vi "PathPlanner_Path_RePlan_Worker2.vi"(4 "StartingPoseTranslation":T1 {"Y" format="%14.3f"; "X" format="%14.3f"}, 5 "in PathPlannerPath":T2 {"AllPoints"."HolonomicRotation"."SIN" format="%13.4f"; "AllPoints"."HolonomicRotation"."COS" format="%13.4f"; "AllPoints"."HolonomicRotation"."VALUE" format="%13.4f"; "AllPoints"."Position"."Y" format="%14.3f"; "AllPoints"."Position"."X" format="%14.3f"; "GoalEndState"."Rotation"."SIN" format="%13.4f"; "GoalEndState"."Rotation"."COS" format="%13.4f"; "GoalEndState"."Rotation"."VALUE" format="%13.4f"; "EventMarkers"."lastRobotPos"."Y" format="%14.3f"; "EventMarkers"."lastRobotPos"."X" format="%14.3f"; "EventMarkers"."markerPos"."Y" format="%14.3f"; "EventMarkers"."markerPos"."X" format="%14.3f"; "RotationTargets"."target"."SIN" format="%13.4f"; "RotationTargets"."target"."COS" format="%13.4f"; "RotationTargets"."target"."VALUE" format="%13.4f"; "PreviewStartingRotation"."SIN" format="%13.4f"; "PreviewStartingRotation"."COS" format="%13.4f"; "PreviewStartingRotation"."VALUE" format="%13.4f"; "BezierPoints"."Y" format="%14.3f"; "BezierPoints"."X" format="%14.3f"}, 6 "robotNextCtrl":T1 {"Y" format="%14.3f"; "X" format="%14.3f"}, 7 "NumPtsMinusOne":i32, 9 "robotNextCtrl_NULL":bool, 10 "ComparePoint":T1 {"Y" format="%14.3f"; "X" format="%14.3f"}, 11 "ClosestDist":dbl) -> (2 "Error":bool, 3 "Replanned Path":T2 {"AllPoints"."HolonomicRotation"."SIN" format="%13.4f"; "AllPoints"."HolonomicRotation"."COS" format="%13.4f"; "AllPoints"."HolonomicRotation"."VALUE" format="%13.4f"; "AllPoints"."Position"."Y" format="%14.3f"; "AllPoints"."Position"."X" format="%14.3f"; "GoalEndState"."Rotation"."SIN" format="%13.4f"; "GoalEndState"."Rotation"."COS" format="%13.4f"; "GoalEndState"."Rotation"."VALUE" format="%13.4f"; "EventMarkers"."lastRobotPos"."Y" format="%14.3f"; "EventMarkers"."lastRobotPos"."X" format="%14.3f"; "EventMarkers"."markerPos"."Y" format="%14.3f"; "EventMarkers"."markerPos"."X" format="%14.3f"; "RotationTargets"."target"."SIN" format="%13.4f"; "RotationTargets"."target"."COS" format="%13.4f"; "RotationTargets"."target"."VALUE" format="%13.4f"; "PreviewStartingRotation"."SIN" format="%13.4f"; "PreviewStartingRotation"."COS" format="%13.4f"; "PreviewStartingRotation"."VALUE" format="%13.4f"; "BezierPoints"."Y" format="%14.3f"; "BezierPoints"."X" format="%14.3f"})   [LabVIEW 2019, in "PathPlanner24.lvlib"]
doc: "Replan path worker 1\n\nNOT COMPLETE. DONT USE."
uses:
  PathPlanner24.lvlib
  TypeDef/PathPlannerPath.ctl
  <vilib>/Rock Robotics/WPI/ThirdParty/JAS_Junk/TrajLib/TypeDef/TRANSLATION2D.ctl
  <vilib>/Rock Robotics/WPI/ThirdParty/JAS_Junk/TrajLib/TypeDef/ROTATION2D.ctl
  TypeDef/PathPlannerRotationTarget.ctl
  TypeDef/PathPlannerConstraintsZone.ctl
  TypeDef/PathPlannerPathConstraints.ctl
  TypeDef/PathPlannerEventMarker.ctl
  TypeDef/PathPlannerCommandUtil.ctl
  ENum/PathPlanner_CommandUtilType_ENUM.ctl
  TypeDef/PathPlannerGoalEndState.ctl
  TypeDef/PathPlannerPathPoint.ctl
  <vilib>/Rock Robotics/WPI/ThirdParty/JAS_Junk/TrajLib/Translation2d_Create.vi
  <vilib>/Rock Robotics/WPI/ThirdParty/JAS_Junk/TrajLib/Translation2d_GetXY.vi
  <vilib>/Rock Robotics/WPI/ThirdParty/JAS_Junk/TrajLib/Rotation2d_CreateXY.vi
  <vilib>/Rock Robotics/WPI/ThirdParty/JAS_Junk/TrajLib/Rotation2d_GetAngleCosSin.vi
  <vilib>/Rock Robotics/WPI/ThirdParty/JAS_Junk/TrajLib/Util_CalcDist.vi
  <vilib>/Rock Robotics/WPI/ThirdParty/JAS_Junk/TrajLib/Trajectory_Library.lvlib
panel:
  # "NOT DONE"
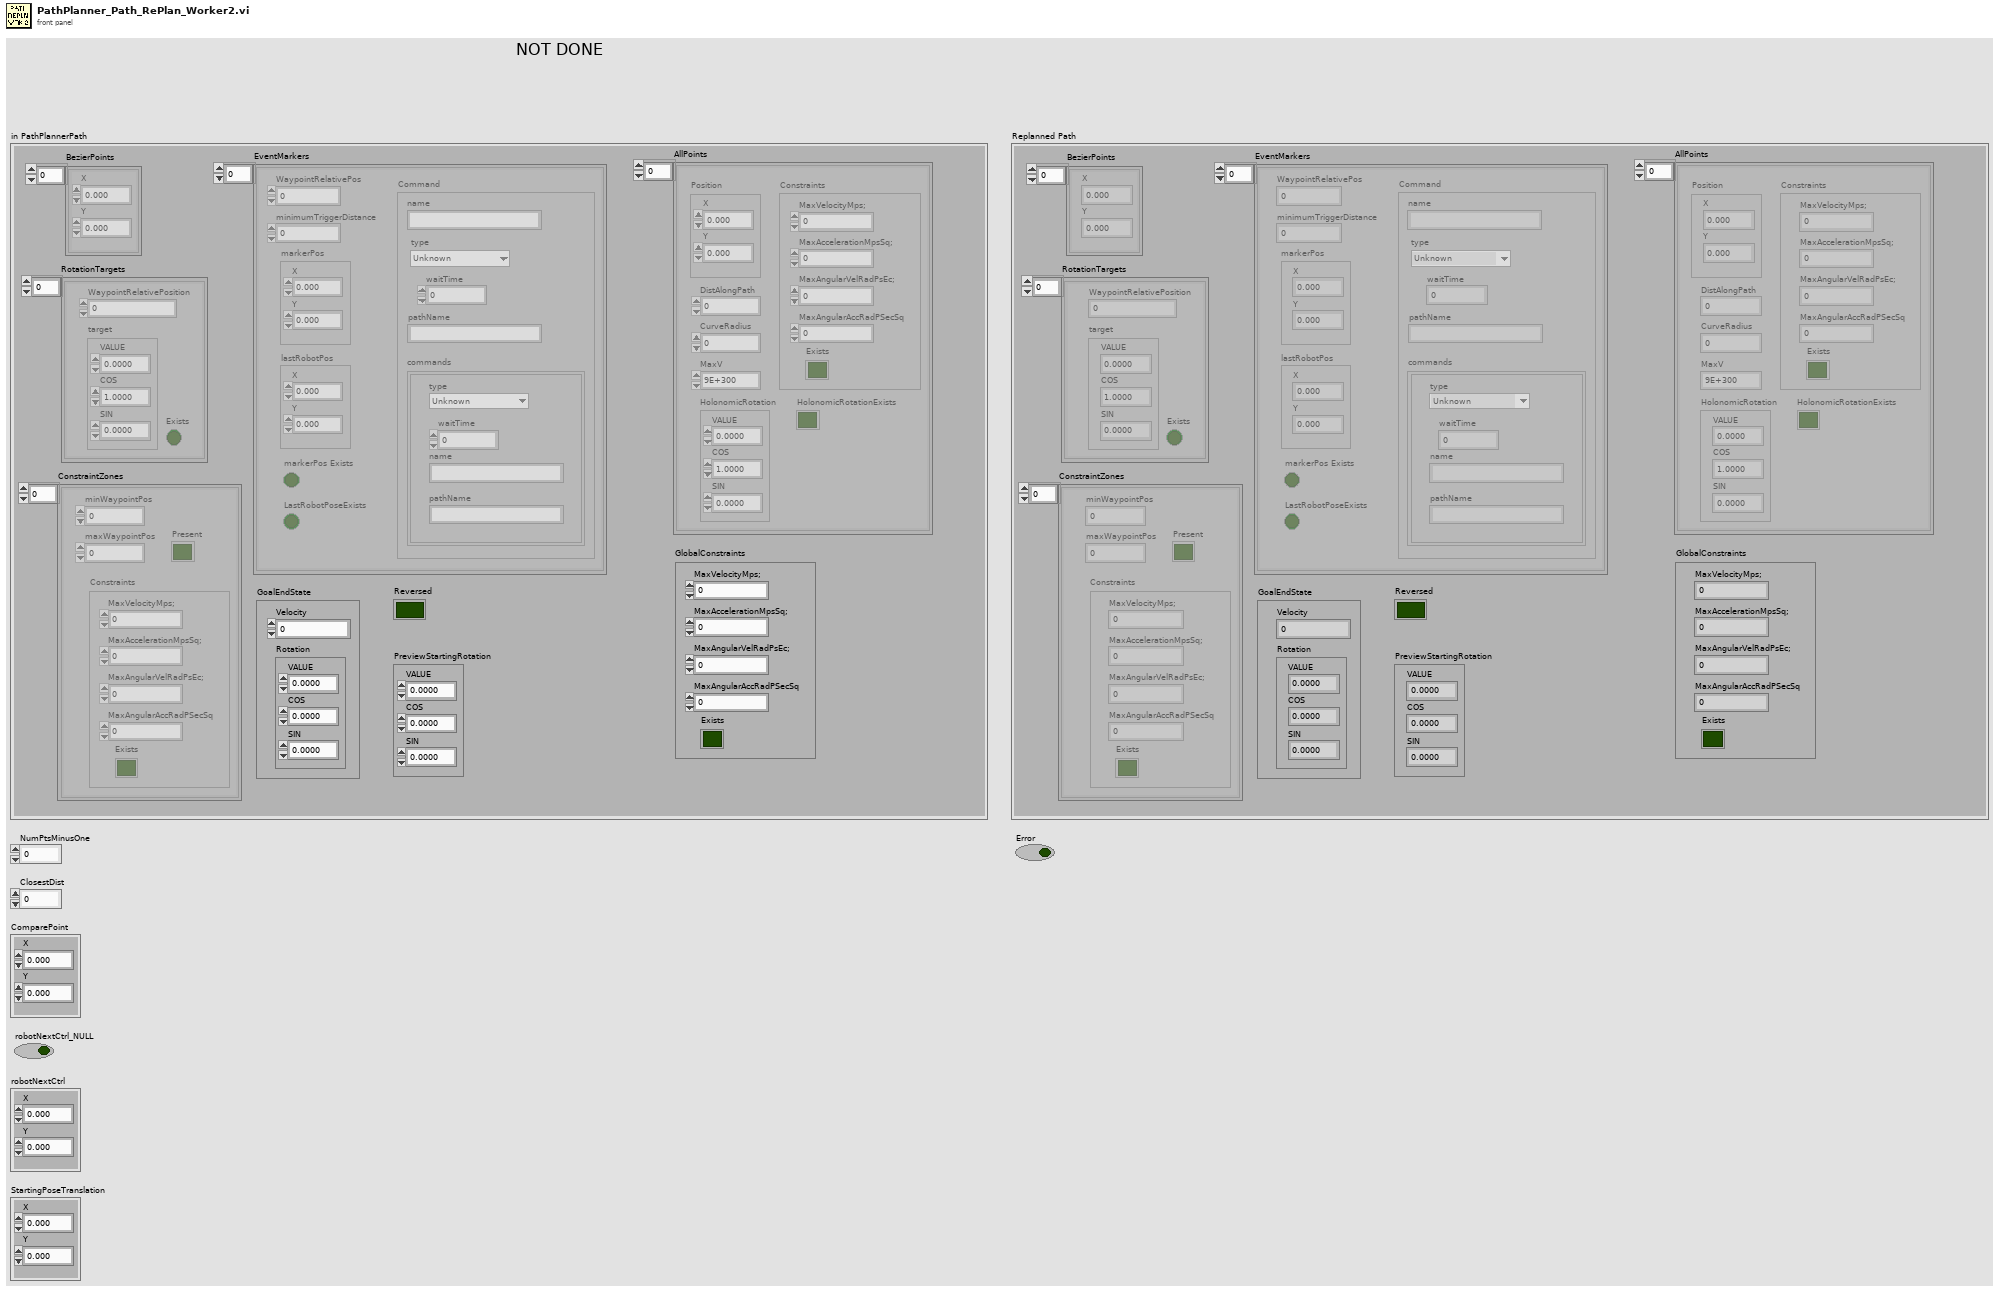
[diagram p1: front panel]
types:
  T1 = typedef "Trajectory_Library.lvlib/TRANSLATION2D.ctl" = cluster{"X":dbl, "Y":dbl}
  T2 = typedef "PathPlanner24.lvlib/PathPlannerPath.ctl" = cluster{"BezierPoints":T1[], "PreviewStartingRotation":T3, "Reversed":bool, "RotationTargets":T4[], "ConstraintZones":T5[], "EventMarkers":T7[], "GlobalConstraints":T6, "GoalEndState":T10, "AllPoints":T11[]}
  T3 = typedef "Trajectory_Library.lvlib/ROTATION2D.ctl" = cluster{"VALUE":dbl, "COS":dbl, "SIN":dbl}
  T4 = typedef "PathPlanner24.lvlib/PathPlannerRotationTarget.ctl" = cluster{"target":T3, "WaypointRelativePosition":dbl, "Exists":bool}
  T5 = typedef "PathPlanner24.lvlib/PathPlannerConstraintsZone.ctl" = cluster{"minWaypointPos":dbl, "maxWaypointPos":dbl, "Constraints":T6, "Present":bool}
  T6 = typedef "PathPlanner24.lvlib/PathPlannerPathConstraints.ctl" = cluster{"MaxVelocityMps;":dbl, "MaxAccelerationMpsSq;":dbl, "MaxAngularVelRadPsEc;":dbl, "MaxAngularAccRadPSecSq":dbl, "Exists":bool}
  T7 = typedef "PathPlanner24.lvlib/PathPlannerEventMarker.ctl" = cluster{"WaypointRelativePos":dbl, "minimumTriggerDistance":dbl, "markerPos":T1, "lastRobotPos":T1, "Command":T8, "markerPos Exists":bool, "LastRobotPoseExists":bool}
  T8 = typedef "PathPlanner24.lvlib/PathPlannerCommandUtil.ctl" = cluster{"waitTime":dbl, "name":string, "pathName":string, "commands":cluster{"type":T9, "waitTime":dbl, "name":string, "pathName":string}[], "type":T9}
  T9 = typedef "PathPlanner24.lvlib/PathPlanner_CommandUtilType_ENUM.ctl" = enum16{"Unknown", "Wait", "Named", "Path", "Sequential", "Parallel", "Race", "Deadline"}
  T10 = typedef "PathPlanner24.lvlib/PathPlannerGoalEndState.ctl" = cluster{"Velocity":dbl, "Rotation":T3}
  T11 = typedef "PathPlanner24.lvlib/PathPlannerPathPoint.ctl" = cluster{"Position":T1, "HolonomicRotation":T3, "DistAlongPath":dbl, "CurveRadius":dbl, "MaxV":dbl, "Constraints":T6, "HolonomicRotationExists":bool}
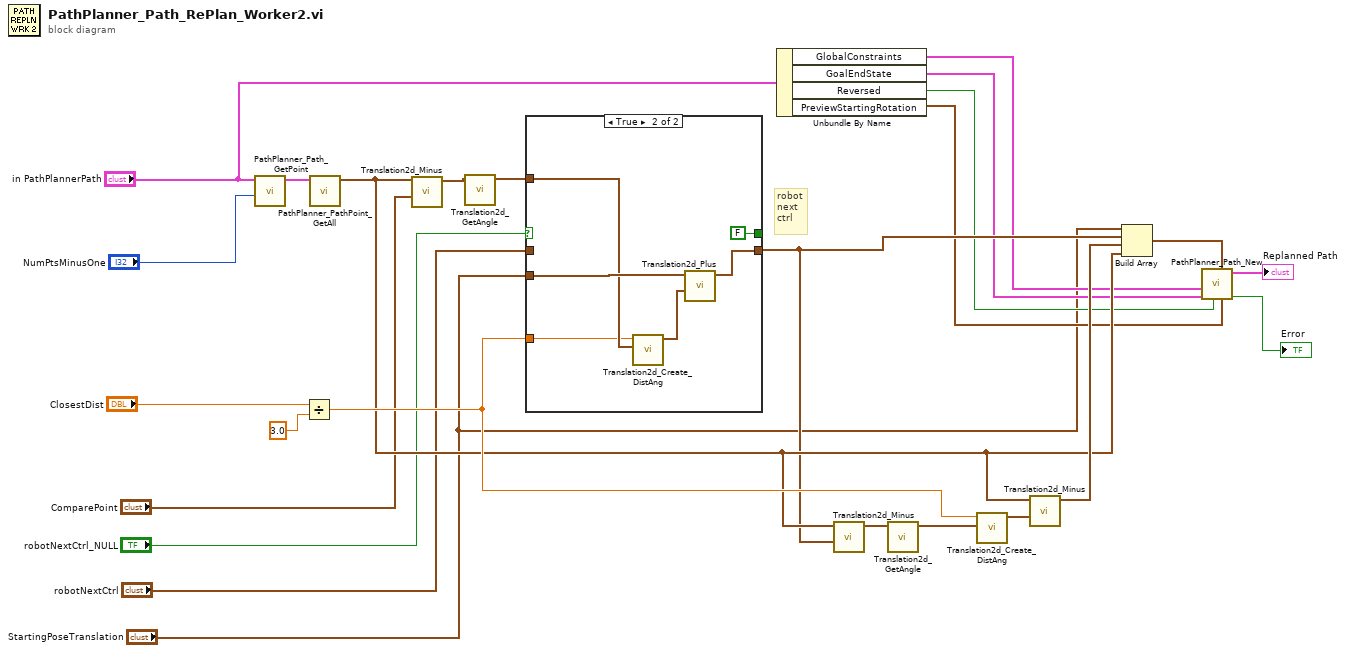
[diagram p0: block diagram]
diagram:
  # "robot\nnext\nctrl"
  n1 = call "PathPlanner_Path_GetPoint.vi"("Index"="NumPtsMinusOne", "PathPlannerPath"="in PathPlannerPath") -> ("Point"=w1:T11)  [unwired: 9 in]
  n2 = Divide(x="ClosestDist", y=3.0) -> (x/y=w24:dbl)
  n3 = call "PathPlanner_PathPoint_GetAll.vi"("PathPlannerPoint"=w1) -> ("Position"=w19:T1)  [unwired: 4 in, 6 out]
  n4 = call <vilib>:"Translation2d_Minus.vi"("other Translation"="ComparePoint", "In Translation"=w19) -> ("Out Translation"=w4:T1)  [unwired: 9 in]
  n5 = call <vilib>:"Translation2d_GetAngle.vi"("In Translation"=w4) -> ("Angle_Rotation2d"=w6:T3)  [unwired: 10 in]
  n6 = case shown="True" "robotNextCtrl_NULL" {
    selector: "robotNextCtrl_NULL" -> [w26 _]
    tunnel: w6 -> [_ w32]
    tunnel: "robotNextCtrl" -> [w27 _]
    tunnel: [w27 w30] -> w17
    tunnel: [w26 FALSE] -> _
    tunnel: "StartingPoseTranslation" -> [_ w33]
    tunnel: w24 -> [_ w28]
    frame False {
    }
    frame True {
      n7 = call <vilib>:"Translation2d_Create_DistAng.vi"("Angle"=w32, "Dist"=w28) -> ("TRANSLATION"=w31:T1)  [unwired: 9 in]
      n8 = call <vilib>:"Translation2d_Plus.vi"("other Translation"=w31, "In Translation"=w33) -> ("Out Translation"=w30:T1)  [unwired: 9 in]
    }
  }
  n9 = Unbundle By Name("in PathPlannerPath") -> ("GlobalConstraints"=w13:T6, "GoalEndState"=w14:T10, "Reversed"=w15:bool, "PreviewStartingRotation"=w16:T3)
  n10 = call <vilib>:"Translation2d_Minus.vi"("other Translation"=w17, "In Translation"=w19) -> ("Out Translation"=w18:T1)  [unwired: 9 in]
  n11 = call <vilib>:"Translation2d_GetAngle.vi"("In Translation"=w18) -> ("Angle_Rotation2d"=w21:T3)  [unwired: 10 in]
  n12 = call <vilib>:"Translation2d_Create_DistAng.vi"("Angle"=w21, "Dist"=w24) -> ("TRANSLATION"=w20:T1)  [unwired: 9 in]
  n13 = call <vilib>:"Translation2d_Minus.vi"("other Translation"=w20, "In Translation"=w19) -> ("Out Translation"=w25:T1)  [unwired: 9 in]
  n14 = Build Array("StartingPoseTranslation", w17, w25, w19) -> (w10:T1[])
  n15 = call "PathPlanner_Path_New.vi"("PreviewStartingRotation"=w16, "BezierPoints"=w10, "Reversed"=w15, "GoalEndState"=w14, "GlobalConstraints"=w13) -> ("Error"=→"Error":bool, "PathPlannerPath"=→"Replanned Path":T2)  [unwired: 5 in]
